vi "Alp Seq Timing.vi"(4 "TriggerInDelay":i32, 5 "SynchPulseWidth":i32, 6 "SynchDelay":i32, 7 "PictureTime":i32, 8 "error in (no error)":errorcluster, 9 "IlluminateTime":i32, 10 "SequenceId":u32, 11 "DeviceId":u32) -> (0 "error out":errorcluster, 3 "function return":i32)   [LabVIEW 2013, in "alpD41.lvlib"]
uses:
  alpD41.lvlib
  alpD41.dll
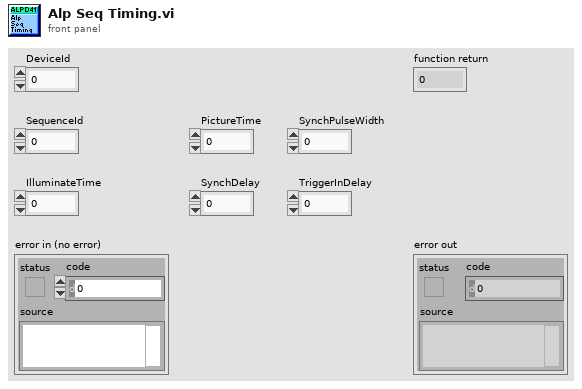
[diagram p1: front panel]
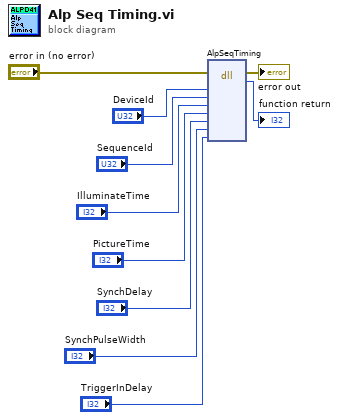
[diagram p0: block diagram]
diagram:
  n1 = dll-call lib="C:/Users/ErNa/Google Drive (ernajqi@gmail.com)/ErNa/LabView/DMD Standalone Codes/Libraries-alpD41/alpD41.*" fn="AlpSeqTiming"(error in="error in (no error)", "DeviceId"="DeviceId", "SequenceId"="SequenceId", "IlluminateTime"="IlluminateTime", "PictureTime"="PictureTime", "SynchDelay"="SynchDelay", "SynchPulseWidth"="SynchPulseWidth", "TriggerInDelay"="TriggerInDelay") -> (error out=→"error out":errorcluster, →"function return":i32)  [unwired: 9 in, 1 out]
